vi "Search Attributes.vi"(7 "Attribute type":refnum<class "Attribute.lvclass">, 10 "[Attributes]":refnum<class "Attribute.lvclass">[](array[class])) -> (1 "found":bool, 2 "Attribute out":refnum<class "Attribute.lvclass">)   [LabVIEW 2019, in "Attribute.lvclass"]
doc: "JKI State Machine Objects (SMO) 1.3.0.56\nJKI - JKI\nCopyright (c) 2017, JKI"
uses:
  Attribute.lvclass
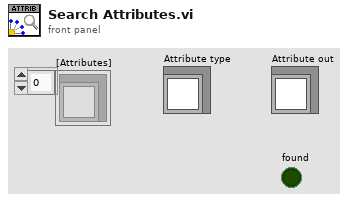
[diagram p1: front panel]
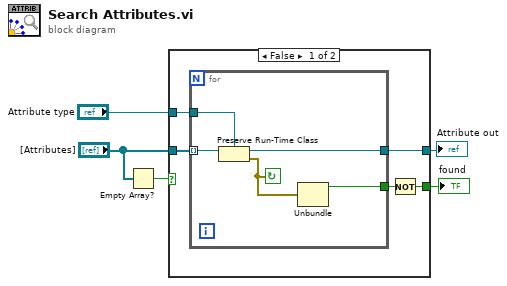
[diagram p0: block diagram]
diagram:
  n1 = Empty Array?(array="[Attributes]") -> (empty?=w1:bool)
  n2 = case shown="False" w1 {
    tunnel: "Attribute type" -> [w10 _]
    tunnel: [w9 _] -> w4
    tunnel: [w7 _] -> w3
    tunnel: "[Attributes]" -> [w6 _]
    frame False {
      n3 = for {
        tunnel: w6 -> [w15] mode=indexing
        tunnel: w10 -> [w14]
        tunnel: [w13] -> w9
        tunnel: [w11] -> w8
        stop <- w12 continue-if-true
        n4 = Preserve Run-Time Class(object in=w15, 2:w14) -> (object out=w13:refnum<class "Attribute.lvclass">, error out=w12:errorcluster)  [unwired: 1 in]
        n5 = Unbundle(w12) -> ("status"=w11:bool)  [unwired: 2 out]
      }
      n6 = Not(x=w8) -> (.not. x?=w7:bool)
    }
    frame True {
    }
  }
  "Attribute out" <- w4
  "found" <- w3
